vi "Pivot Module.vi"(0 "pivot":enum16{"FL", "FR", "BL", "BR"}(ring)) -> ()   [LabVIEW 2014]
uses:
  <vilib>/Rock Robotics/WPI/SafetyOutput/WPI_SafetyOutputConfigMenu.ctl
  Begin/Global RefNums.vi
  Begin/Global Variables.vi
  Begin/Global Constants.vi
panel:
  out "s? t:f":dbl
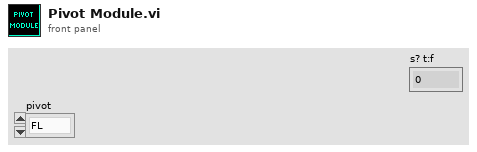
[diagram p1: front panel]
types:
  T1 = typedef "WPI_SafetyOutputConfigMenu.ctl" = enum16{"Enable", "Disable"}
  T2 = typedef "WPI_AnalogChannelDevRef.ctl" = cluster{"DevStatus":errorcluster, "Controller":T3, "Analog Channel":T4}
  T3 = typedef "FPGA_TypedefAnalogModule.ctl" = enum16{"Controller 1"}
  T4 = typedef "FPGA_AIChannel.ctl" = enum8{"AI 0", "AI 1", "AI 2", "AI 3", "AI MXP 0", "AI MXP 1", "AI MXP 2", "AI MXP 3", "Invalid"}
  T5 = typedef "WPI_MotorControlDeviceRef.ctl" = cluster{"DeviceStatus":errorcluster, "Type":T6, "PWM":cluster{"Controller":T7, "PWM Channel":T8, "DeadBand":T9}, "CAN":cluster{"Device Number":u8, "Control Mode":T10, "Semaphore":T11, "Max Vout":dbl, "TalonSRX Control Mode":T12}, "Invert":bool, "TransformRef":T13, "InvTransformRef":T13}
  T6 = typedef "WPI_MotorControlType.ctl" = enum16{"PWM", "CAN", "CANTalonSRX"}
  T7 = typedef "FPGA_TypedefDigitalModule.ctl" = enum16{"Controller 1"}
  T8 = typedef "FPGA_DIOPWMChannel.ctl" = enum8{"PWM 0", "PWM 1", "PWM 2", "PWM 3", "PWM 4", "PWM 5", "PWM 6", "PWM 7", "PWM 8", "PWM 9", "PWM MXP 0", "PWM MXP 1", "PWM MXP 2", "PWM MXP 3", "PWM MXP 4", "PWM MXP 5", "PWM MXP 6", "PWM MXP 7", "PWM MXP 8", "PWM MXP 9", "Invalid"}
  T9 = typedef "WPI_PWMDeadband.ctl" = cluster{"Name":string, "maxPositivePwm":i32, "minPositivePwm":i32, "centerPwm":i32, "maxNegativePwm":i32, "minNegativePwm":i32, "angularRange":u16}
  T10 = typedef "WPI_CANJaguar_ControlMode.ctl" = enum8{"Percent VBus", "Current", "Speed", "Position", "Voltage"}
  T11 = typedef "Semaphore RefNum" = refnum<k1>
  T12 = typedef "WPI_CANTalonSRX_APIControlMode.ctl" = enum8{"Percent VBus", "Speed", "Position", "Slave", "Unchanged / Invalid"}
  T13 = typedef "WPI_PWMTransform_ConPane.ctl" = refnum<vi>
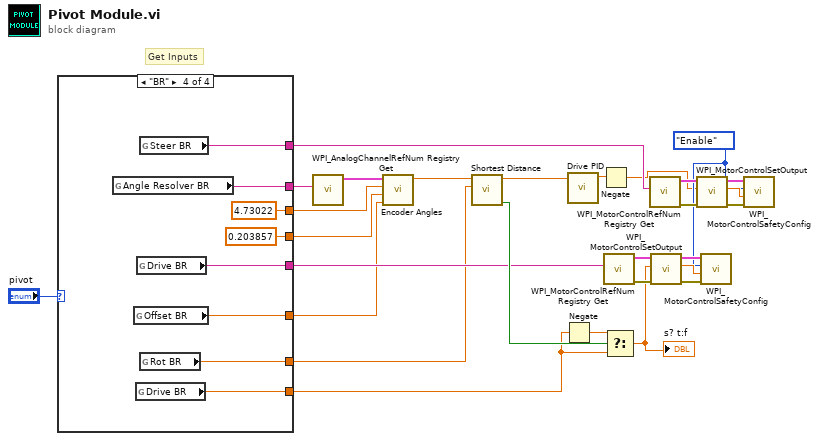
[diagram p0: block diagram]
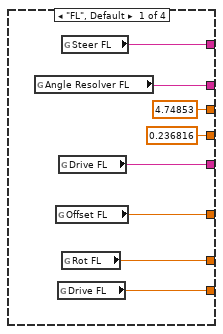
[diagram p2: hidden frame]
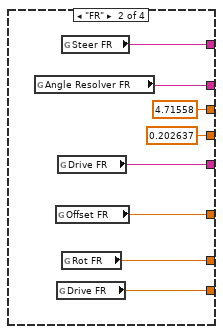
[diagram p3: hidden frame]
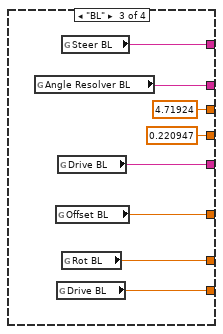
[diagram p4: hidden frame]
diagram:
  w15 = WPI_SafetyOutputConfigMenu."Enable" ("mode")
  # "Get Inputs"
  n1 = case shown="\"BR\"" "pivot" {
    tunnel: [w36 w44 w52 w60] -> w10
    tunnel: [w35 w43 w51 w59] -> w9
    tunnel: [w34 w42 w50 w58] -> w8
    tunnel: [w33 w41 w49 w57] -> w7
    tunnel: [w32 w40 w48 w56] -> w6
    tunnel: [w31 w39 w47 w55] -> w5
    tunnel: [4.74853 ("Resolver BL High Voltage") 4.71558 ("Resolver BL High Voltage") 4.71924 ("Resolver BL High Voltage") 4.73022 ("Resolver BL High Voltage")] -> w4
    tunnel: [0.236816 ("Resolver BL Low Voltage") 0.202637 ("Resolver BL Low Voltage") 0.220947 ("Resolver BL Low Voltage") 0.203857 ("Resolver BL Low Voltage")] -> w3
    frame "FL", Default {
      n2 = global read "Global RefNums.vi" "Angle Resolver FL"() -> (w35:string)
      n3 = global read "Global Constants.vi" "Offset FL"() -> (w33:dbl)
      n4 = global read "Global Variables.vi" "Drive FL"() -> (w31:dbl)
      n5 = global read "Global RefNums.vi" "Drive FL"() -> (w34:string)
      n6 = global read "Global RefNums.vi" "Steer FL"() -> (w36:string)
      n7 = global read "Global Variables.vi" "Rot FL"() -> (w32:dbl)
    }
    frame "FR" {
      n8 = global read "Global RefNums.vi" "Angle Resolver FR"() -> (w43:string)
      n9 = global read "Global Constants.vi" "Offset FR"() -> (w41:dbl)
      n10 = global read "Global Variables.vi" "Drive FR"() -> (w39:dbl)
      n11 = global read "Global RefNums.vi" "Drive FR"() -> (w42:string)
      n12 = global read "Global RefNums.vi" "Steer FR"() -> (w44:string)
      n13 = global read "Global Variables.vi" "Rot FR"() -> (w40:dbl)
    }
    frame "BL" {
      n14 = global read "Global RefNums.vi" "Angle Resolver BL"() -> (w51:string)
      n15 = global read "Global Constants.vi" "Offset BL"() -> (w49:dbl)
      n16 = global read "Global Variables.vi" "Drive BL"() -> (w47:dbl)
      n17 = global read "Global RefNums.vi" "Drive BL"() -> (w50:string)
      n18 = global read "Global RefNums.vi" "Steer BL"() -> (w52:string)
      n19 = global read "Global Variables.vi" "Rot BL"() -> (w48:dbl)
    }
    frame "BR" {
      n20 = global read "Global RefNums.vi" "Angle Resolver BR"() -> (w59:string)
      n21 = global read "Global Constants.vi" "Offset BR"() -> (w57:dbl)
      n22 = global read "Global Variables.vi" "Drive BR"() -> (w55:dbl)
      n23 = global read "Global RefNums.vi" "Drive BR"() -> (w58:string)
      n24 = global read "Global RefNums.vi" "Steer BR"() -> (w60:string)
      n25 = global read "Global Variables.vi" "Rot BR"() -> (w56:dbl)
    }
  }
  n26 = call <vilib>:"WPI_AnalogChannelRefNum Registry Get.vi"("refnum name"=w9) -> ("AIDeviceRef"=w28:T2)  [unwired: 9 in, 1 out]
  n27 = call "Encoder Angles.vi"("calibration angle"=w7, "low voltage"=w3, "top voltage"=w4, "AIDeviceRef Encoder"=w28) -> ("encoder angle"=w27:dbl)  [unwired: 7 in]
  n28 = call "Shortest Distance.vi"("target"=w6, "current"=w27) -> ("flipping?"=w12:bool, "angle to rotate"=w26:dbl)  [unwired: 8 in]
  n29 = Negate(x=w5) -> (-x=w13:dbl)
  n30 = call "Drive PID.vi"("Process Variable"=w26) -> ("Output"=w2:dbl)  [unwired: 10 in]
  n31 = Negate(x=w2) -> (-x=w1:dbl)
  n32 = call <vilib>:"WPI_MotorControlRefNum Registry Get.vi"("refnum name"=w8) -> ("error out"=w20:errorcluster, "MotorControlDevRef"=w19:T5)  [unwired: 9 in]
  n33 = Select(t=w13, s=w12, f=w5) -> (s? t:f=w14:dbl)
  "s? t:f" <- w14
  n34 = call <vilib>:"WPI_MotorControlRefNum Registry Get.vi"("refnum name"=w10) -> ("error out"=w25:errorcluster, "MotorControlDevRef"=w24:T5)  [unwired: 9 in]
  n35 = call <vilib>:"WPI_MotorControlSetOutput.vi"("error in (no error)"=w20, "Output"=w14, "MotorControlDevRef"=w19) -> ("error out"=w18:errorcluster, "Motor Output"=w17:dbl, "MotorControlDevRef"=w16:T5)  [unwired: 6 in]
  n36 = call <vilib>:"WPI_MotorControlSetOutput.vi"("error in (no error)"=w25, "Output"=w1, "MotorControlDevRef"=w24) -> ("error out"=w23:errorcluster, "Motor Output"=w22:dbl, "MotorControlDevRef"=w21:T5)  [unwired: 6 in]
  n37 = call <vilib>:"WPI_MotorControlSafetyConfig.vi"("error in (no error)"=w18, "timeout (s)"=w17, "mode"=w15, "MotorControlDevRef"=w16) -> ()  [unwired: 6 in, 2 out]
  n38 = call <vilib>:"WPI_MotorControlSafetyConfig.vi"("error in (no error)"=w23, "timeout (s)"=w22, "mode"=w15, "MotorControlDevRef"=w21) -> ()  [unwired: 6 in, 2 out]
